vi "String Is Numeric.vi"(2 "scan format (%.;%e)":string="%.;%e", 3 "String":string) -> (0 "Numeric":dbl, 1 "is numeric":bool)   [LabVIEW 2013]
doc: "Detects if the String is pure numeric. If it contains some rubbish after or before number it will be non-numeric."
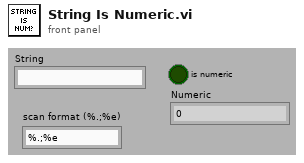
[diagram p1: front panel]
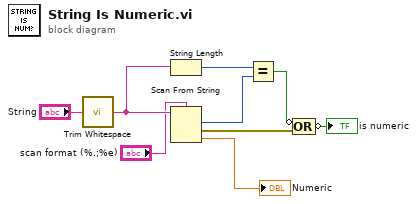
[diagram p0: block diagram]
diagram:
  n1 = call <vilib>:"Trim Whitespace.vi"("string"="String") -> ("trimmed string"=w7:string)  [unwired: 1 in]
  n2 = String Length(string=w7) -> (length=w6:i32)
  n3 = Scan From String(format string="scan format (%.;%e)", input string=w7) -> (offset past scan=w5:u32, error out=w3:errorcluster, output 1=→"Numeric":dbl)  [unwired: 3 in, 1 out]
  n4 = Equal?(x=w6, y=w5) -> (x = y?=w4:bool)
  n5 = Compound Arithmetic op=OR(invert w4, w3) -> (invert →"is numeric":bool)
